vi "GEOM_Line2Overrwcs.vi"(6 "curr mult array":string[][][](array[string]), 9 "curr arr":string[][](array[string]), 10 "extension data":string) -> (1 "mout":string[][][](array[string]), 2 "out":string[][](array[string]))   [LabVIEW 2016]
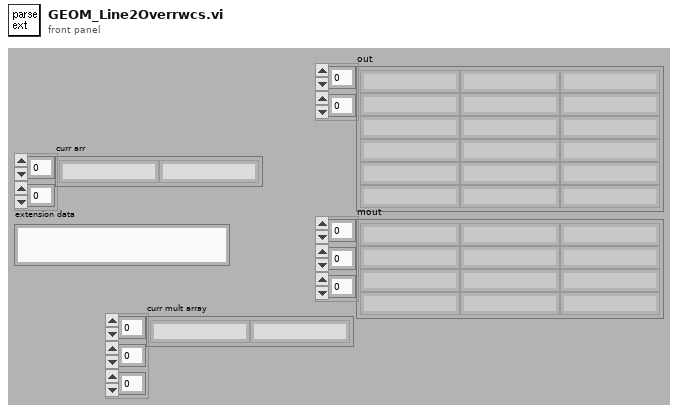
[diagram p1: front panel]
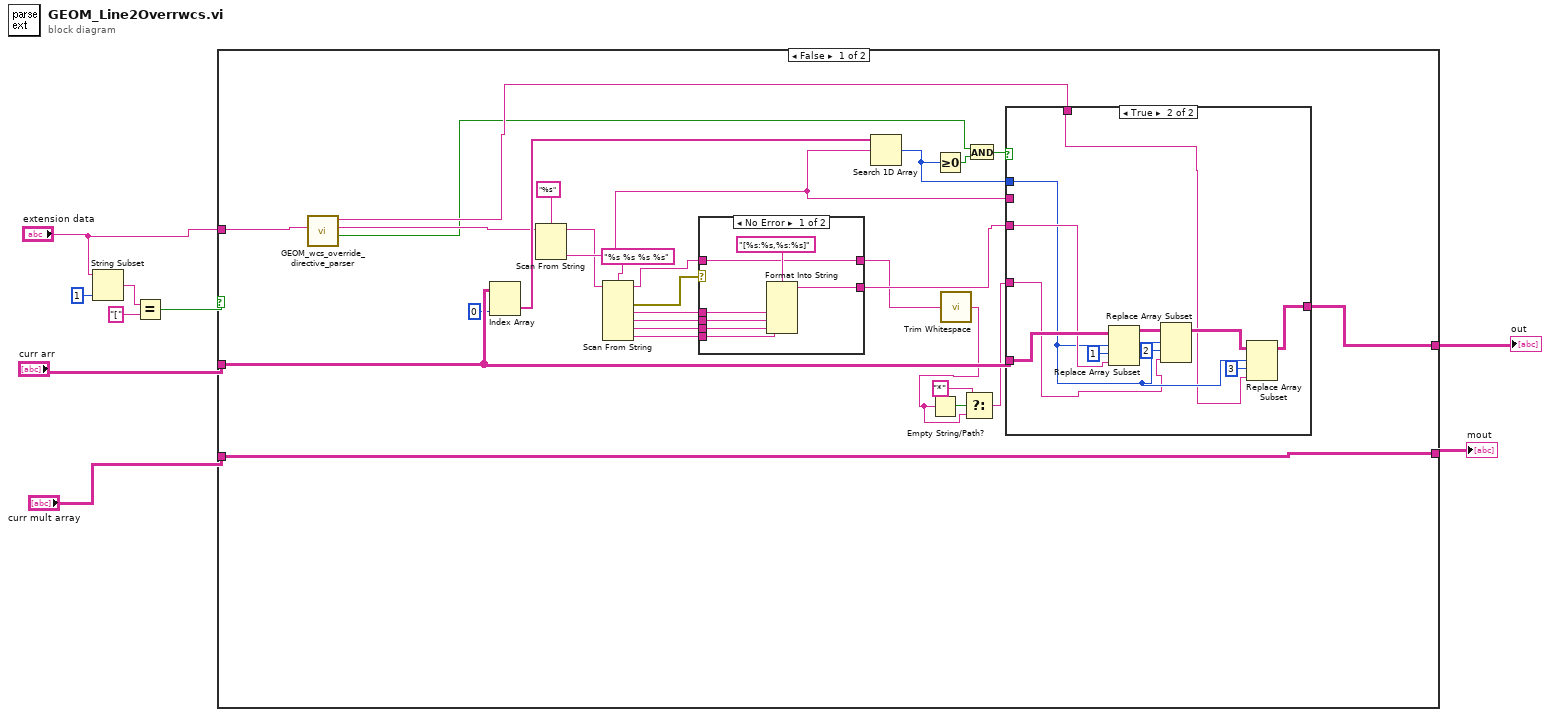
[diagram p0: block diagram]
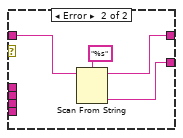
[diagram p2: hidden frame]
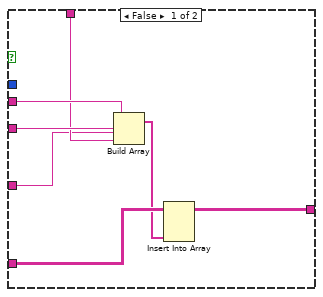
[diagram p3: hidden frame]
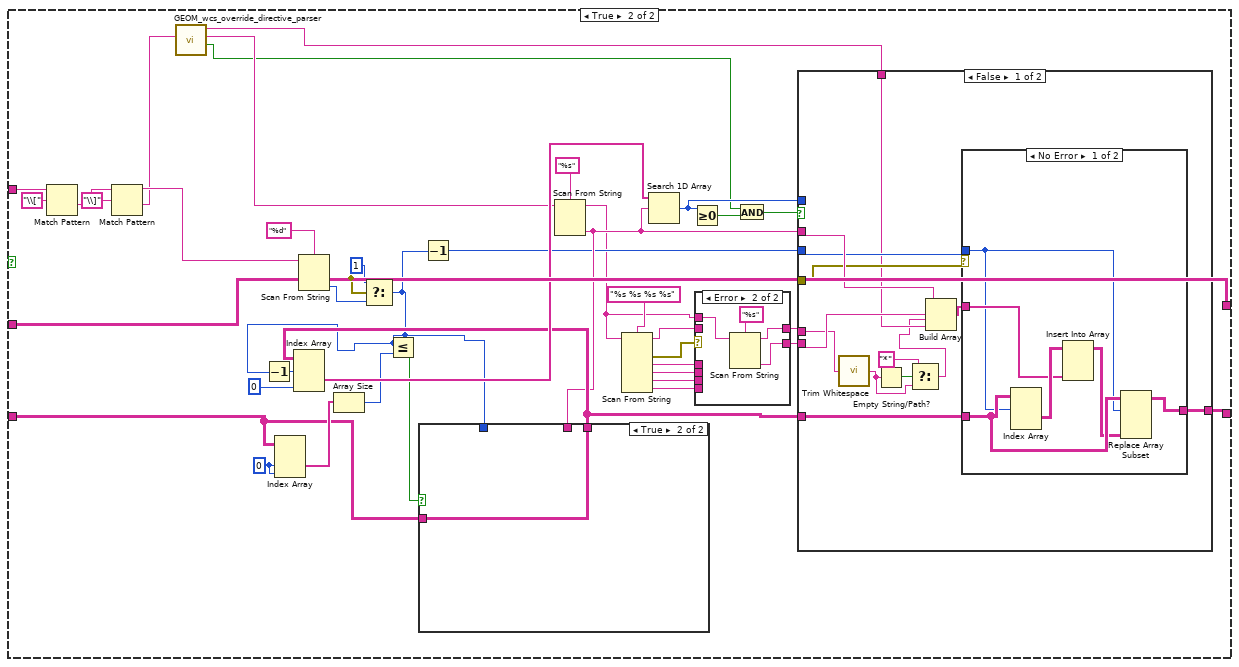
[diagram p4: hidden frame]
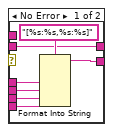
[diagram p5: hidden frame]
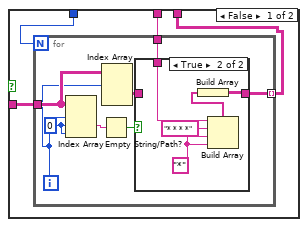
[diagram p6: hidden frame]
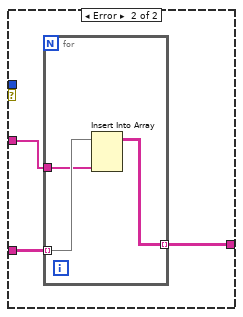
[diagram p8: hidden frame]
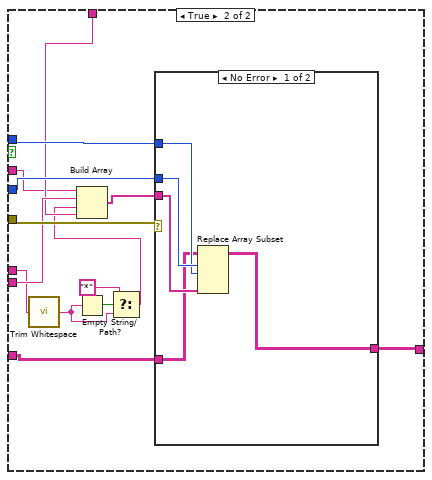
[diagram p9: hidden frame]
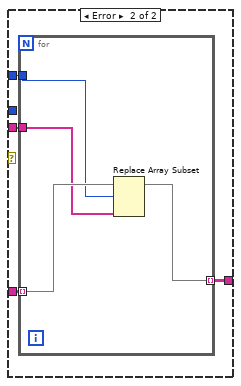
[diagram p10: hidden frame]
diagram:
  n1 = String Subset(string="extension data", length (rest)=1 ("length (rest)")) -> (substring=w6:string)  [unwired: 1 out]
  n2 = Equal?(x=w6, y="[") -> (x = y?=w4:bool)
  n3 = case shown="False" w4 {
    tunnel: [w37 w103] -> w9
    tunnel: "curr arr" -> [w36 w103]
    tunnel: "extension data" -> [w16 w107]
    tunnel: "curr mult array" -> [w24 w86]
    tunnel: [w24 w92] -> w2
    frame False {
      n4 = call "GEOM_wcs_override_directive_parser.vi"("modif in"=w16) -> ("override?"=w11:bool, "modif out"=w15:string, "last col"=w14:string)  [unwired: 8 out]
      n5 = Index Array(array=w36, index (col)=0 ("disabled index (col)")) -> (element=w35:string[])  [unwired: 1 in]
      n6 = Scan From String(format string="%s", input string=w15) -> (remaining string=w17:string, output 1=w31:string)  [unwired: 2 in, 3 out]
      n7 = Scan From String(format string="%s %s %s %s", input string=w17) -> (remaining string=w10:string, error out=w23:errorcluster, output 1=w29:string, output 2=w28:string, output 3=w27:string, output 4=w26:string)  [unwired: 2 in, 5 out]
      n8 = case shown="No Error" w23 {
        tunnel: w29 -> [w43 _]
        tunnel: w28 -> [w42 _]
        tunnel: w27 -> [w41 _]
        tunnel: w26 -> [w40 _]
        tunnel: [w39 w46] -> w25
        tunnel: w10 -> [w38 w45]
        tunnel: [w38 w48] -> w20
        frame No Error {
          n9 = Format Into String(format string="[%s:%s,%s:%s]", w43, w42, w41, w40) -> (resulting string=w39:string)  [unwired: 2 in, 1 out]
        }
        frame Error {
          n10 = Scan From String(format string="%s", input string=w45) -> (remaining string=w48:string, output 1=w46:string)  [unwired: 2 in, 3 out]
        }
      }
      n11 = Search 1D Array(1D array=w35, element=w31) -> (index of element=w33:i32)  [unwired: 1 out]
      n12 = Greater Or Equal To 0?(x=w33) -> (x >= 0?=w13:bool)
      n13 = call <vilib>:"Trim Whitespace.vi"("string"=w20) -> ("trimmed string"=w18:string)  [unwired: 1 in]
      n14 = Empty String/Path?(string/path=w18) -> (empty?=w21:bool)
      n15 = Select(t="*", s=w21, f=w18) -> (s? t:f=w19:string)
      n16 = And(x=w11, y=w13) -> (x .and. y?=w12:bool)
      n17 = case shown="True" w12 {
        tunnel: w25 -> [w51 w64]
        tunnel: w31 -> [w52 _]
        tunnel: w36 -> [w55 w66]
        tunnel: [w53 w57] -> w37
        tunnel: w33 -> [_ w60]
        tunnel: w19 -> [w49 w56]
        tunnel: w14 -> [w50 w58]
        frame False {
          n18 = Build Array(w52, w51, w49, w50) -> (w54:string[])
          n19 = Insert Into Array(array=w55, new element=w54) -> (w53:string[][])  [unwired: 2 in]
        }
        frame True {
          n20 = Replace Array Subset(array=w66, new element=w64, index (row)=w60, index (col)=1 ("disabled index (col)")) -> (w63:string[][])
          n21 = Replace Array Subset(array=w63, new element=w56, index (row)=w60, index (col)=2 ("disabled index (col)")) -> (w61:string[][])
          n22 = Replace Array Subset(array=w61, new element=w58, index (row)=w60, index (col)=3 ("disabled index (col)")) -> (w57:string[][])
        }
      }
    }
    frame True {
      w89 = 0 ("disabled index (row)")
      n23 = Match Pattern(string=w107, regular expression="\\[") -> (after substring=w105:string)  [unwired: 4 out]
      n24 = Match Pattern(string=w105, regular expression="\\]") -> (before substring=w73:string, after substring=w70:string)  [unwired: 3 out]
      n25 = call "GEOM_wcs_override_directive_parser.vi"("modif in"=w70) -> ("override?"=w67:bool, "modif out"=w72:string, "last col"=w71:string)  [unwired: 8 out]
      n26 = Index Array(array=w86, index (dim 1)=w89, index (dim 2)=w89) -> (element=w90:string[])  [unwired: 1 in]
      n27 = Scan From String(format string="%d", input string=w73) -> (error out=w81:errorcluster, output 1=w79:i32)  [unwired: 2 in, 3 out]
      n28 = Array Size(array=w90) -> (size(s)=w88:i32)
      n29 = Select(t=1, s=w81, f=w79) -> (s? t:f=w78:i32)
      n30 = Decrement(x=w78) -> (x-1=w84:i32)
      n31 = Less Or Equal?(x=w78, y=w88) -> (x <= y?=w87:bool)
      n32 = Decrement(x=w78) -> (x-1=w82:i32)
      n33 = Scan From String(format string="%s", input string=w72) -> (remaining string=w76:string, output 1=w83:string)  [unwired: 2 in, 3 out]
      n34 = case shown="True" w87 {
        tunnel: w86 -> [w122 w137]
        tunnel: [w121 w137] -> w85
        tunnel: w78 -> [w120 _]
        tunnel: w83 -> [w119 _]
        frame False {
          n35 = for {
            N: w120 -> [_]
            tunnel: w122 -> [w127]
            tunnel: [w124] -> w121 mode=indexing
            tunnel: w119 -> [w123]
            i -> [w126]
            w130 = 0 ("disabled index (row)")
            n36 = Index Array(array=w127, index (dim 0)=w126, index (dim 1)=w130, index (dim 2)=w130) -> (element=w129:string)
            n37 = Empty String/Path?(string/path=w129) -> (empty?=w128:bool)
            n38 = Index Array(array=w127, index (dim 0)=w126) -> (element=w125:string[][])  [unwired: 2 in]
            n39 = case shown="True" w128 {
              tunnel: w125 -> [w131 _]
              tunnel: [w131 w134] -> w124
              tunnel: w123 -> [_ w136]
              frame False {
              }
              frame True {
                w132 = "*" ("element")
                n40 = Build Array(w136, "* * * *" ("element"), w132, w132) -> (w135:string[])
                n41 = Build Array(w135) -> (w134:string[][])
              }
            }
          }
        }
        frame True {
        }
      }
      n42 = Index Array(array=w85, index (dim 0)=w84, index (dim 2)=0 ("disabled index (col)")) -> (element=w99:string[])  [unwired: 1 in]
      n43 = Scan From String(format string="%s %s %s %s", input string=w76) -> (remaining string=w75:string, error out=w77:errorcluster, output 1=w98:string, output 2=w97:string, output 3=w96:string, output 4=w95:string)  [unwired: 2 in, 5 out]
      n44 = Search 1D Array(1D array=w99, element=w83) -> (index of element=w91:i32)  [unwired: 1 out]
      n45 = Greater Or Equal To 0?(x=w91) -> (x >= 0?=w69:bool)
      n46 = case shown="Error" w77 {
        tunnel: w98 -> [w113 _]
        tunnel: w97 -> [w112 _]
        tunnel: w96 -> [w111 _]
        tunnel: w95 -> [w110 _]
        tunnel: [w109 w116] -> w93
        tunnel: w76 -> [_ w118]
        tunnel: w75 -> [w108 _]
        tunnel: [w108 w115] -> w74
        frame No Error {
          n47 = Format Into String(format string="[%s:%s,%s:%s]", w113, w112, w111, w110) -> (resulting string=w109:string)  [unwired: 2 in, 1 out]
        }
        frame Error {
          n48 = Scan From String(format string="%s", input string=w118) -> (remaining string=w115:string, output 1=w116:string)  [unwired: 2 in, 3 out]
        }
      }
      n49 = And(x=w67, y=w69) -> (x .and. y?=w68:bool)
      n50 = case shown="False" w68 {
        tunnel: w74 -> [w148 w166]
        tunnel: w83 -> [w150 w163]
        tunnel: w93 -> [w149 w173]
        tunnel: w85 -> [w145 w175]
        tunnel: w81 -> [w147 w176]
        tunnel: [w144 w171] -> w92
        tunnel: w82 -> [w143 w170]
        tunnel: w91 -> [_ w174]
        tunnel: w71 -> [w142 w169]
        frame False {
          n51 = call <vilib>:"Trim Whitespace.vi"("string"=w148) -> ("trimmed string"=w138:string)  [unwired: 1 in]
          n52 = Empty String/Path?(string/path=w138) -> (empty?=w140:bool)
          n53 = Select(t="*", s=w140, f=w138) -> (s? t:f=w139:string)
          n54 = Build Array(w150, w149, w139, w142) -> (w146:string[])
          n55 = case shown="No Error" w147 {
            tunnel: w146 -> [w155 w158]
            tunnel: w145 -> [w154 w159]
            tunnel: [w151 w157] -> w144
            tunnel: w143 -> [w153 _]
            frame No Error {
              n56 = Index Array(array=w154, index (dim 0)=w153) -> (element=w156:string[][])  [unwired: 2 in]
              n57 = Insert Into Array(array=w156, new element=w155) -> (w152:string[][])  [unwired: 2 in]
              n58 = Replace Array Subset(array=w154, new element=w152, index (dim 0)=w153) -> (w151:string[][][])  [unwired: 2 in]
            }
            frame Error {
              n59 = for {
                tunnel: w159 -> [w162] mode=indexing
                tunnel: w158 -> [w161]
                tunnel: [w160] -> w157 mode=indexing
                n60 = Insert Into Array(array=w162, new element=w161) -> (w160:string[][])  [unwired: 2 in]
              }
            }
          }
        }
        frame True {
          n61 = call <vilib>:"Trim Whitespace.vi"("string"=w166) -> ("trimmed string"=w165:string)  [unwired: 1 in]
          n62 = Empty String/Path?(string/path=w165) -> (empty?=w167:bool)
          n63 = Select(t="*", s=w167, f=w165) -> (s? t:f=w164:string)
          n64 = Build Array(w163, w173, w164, w169) -> (w172:string[])
          n65 = case shown="No Error" w176 {
            tunnel: w175 -> [w177 w185]
            tunnel: w174 -> [w178 w184]
            tunnel: w172 -> [w179 w183]
            tunnel: [w181 w182] -> w171
            tunnel: w170 -> [w180 _]
            frame No Error {
              n66 = Replace Array Subset(array=w177, new element=w179, index (dim 0)=w180, index (dim 1)=w178) -> (w181:string[][][])  [unwired: 1 in]
            }
            frame Error {
              n67 = for {
                tunnel: w185 -> [w189] mode=indexing
                tunnel: w184 -> [w188]
                tunnel: w183 -> [w187]
                tunnel: [w186] -> w182 mode=indexing
                n68 = Replace Array Subset(array=w189, new element=w187, index (row)=w188) -> (w186:string[][])  [unwired: 1 in]
              }
            }
          }
        }
      }
    }
  }
  "out" <- w9
  "mout" <- w2
